vi "test2.vi"() -> ()   [LabVIEW 2018]
uses:
  #include/Global Variables.vi
panel:
  out "JSON string":string
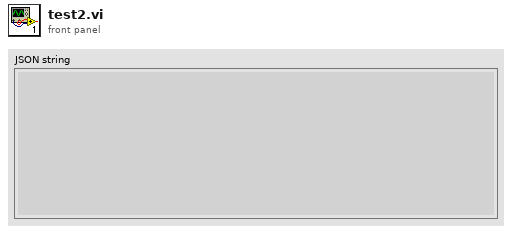
[diagram p1: front panel]
types:
  T1 = cluster{"jsonGen":string[], "jsonGen 2":string[]}
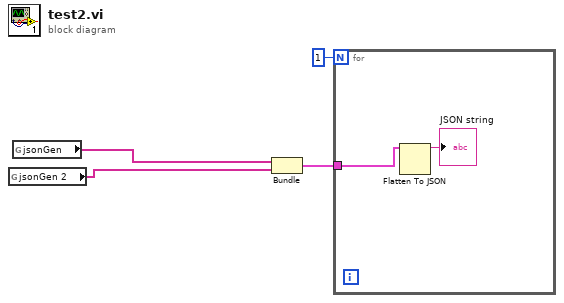
[diagram p0: block diagram]
diagram:
  n1 = global read "Global Variables.vi" "jsonGen 2"() -> (w2:string[])
  n2 = global read "Global Variables.vi" "jsonGen"() -> (w4:string[])
  n3 = Bundle("jsonGen"=w4, "jsonGen 2"=w2) -> (w3:T1)  [unwired: 1 in]
  n4 = for {
    N: 1 -> [_]
    tunnel: w3 -> [w5]
    n5 = Flatten To JSON(anything=w5) -> (JSON string=→"JSON string":string)  [unwired: 2 in, 1 out]
  }
